vi "XYZStage-Reset axis command.vi"(8 "error in (no error)":errorcluster, 9 "XYZ Stage dequeued data":T2={"Command"=enum."Initialize", "Channel"="Z", "X"=0.0, "Y"=0.0, "Z"=0.0, "Speed"=0, "Zero"=FALSE, "Use acknowledgement?"=TRUE} {"Speed" format="Speed= %.0f"; "Z" format="Z= %#_g"; "Y" format="Y= %#_g"; "X" format="X= %#_g"}, 10 "Z Stage":T1, 11 "XY Stage":T5) -> (0 "error out":errorcluster)   [LabVIEW 2020]
uses:
  Typedefs/XY Stage config cluster.ctl
  Typedefs/XYZ stage data.ctl
  Typedefs/XYZ stage states.ctl
  Typedefs/XYZ channel ring.ctl
  Typedefs/Z Stage config cluster.ctl
  Global Variables/General Globals.vi
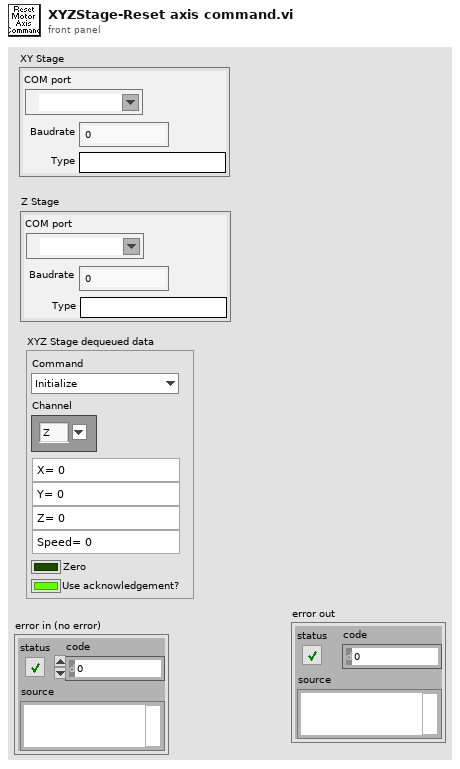
[diagram p1: front panel]
types:
  T1 = typedef "Z Stage config cluster.ctl" = cluster{"COM port":refnum<visa-resource-name>, "Baudrate":i32, "Type":string}
  T2 = typedef "XYZ stage data.ctl" = cluster{"Command":T3, "Channel":T4, "X":sgl, "Y":sgl, "Z":sgl, "Speed":i32, "Zero":bool, "Use acknowledgement?":bool}
  T3 = typedef "XYZ stage states.ctl" = enum16{"Dequeue", "Initialize", "Read Position", "Read Speed Setting", "Move", "Set Max Speed", "Reset Axis", "Stop all movement"}
  T4 = typedef "XYZ channel ring.ctl" = string
  T5 = typedef "XY Stage config cluster.ctl" = cluster{"COM port":refnum<visa-resource-name>, "Baudrate":i32, "Type":string}
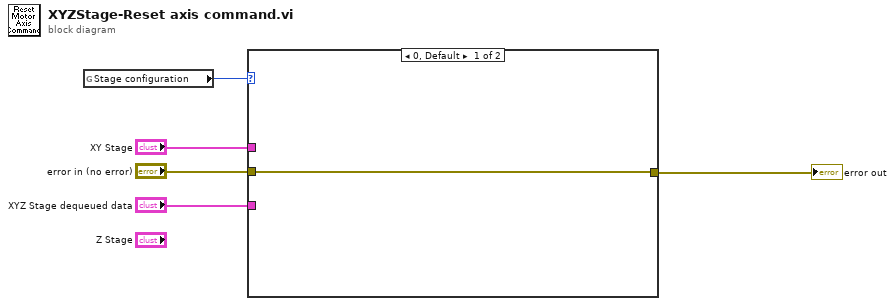
[diagram p0: block diagram]
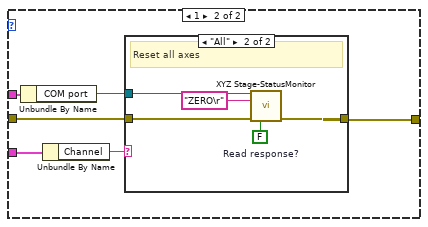
[diagram p2: hidden frame]
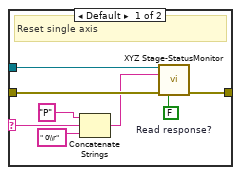
[diagram p3: hidden frame]
diagram:
  n1 = global read "General Globals.vi" "Stage configuration"() -> (w1:i32)
  n2 = case shown="0, Default" w1 {
    tunnel: [w6 w12] -> w5
    tunnel: "XYZ Stage dequeued data" -> [_ w11]
    tunnel: "error in (no error)" -> [w6 w9]
    tunnel: "XY Stage" -> [_ w8]
    frame 0, Default {
    }
    frame 1 {
      n3 = Unbundle By Name(w8) -> ("COM port"=w7:refnum<visa-resource-name>)
      n4 = Unbundle By Name(w11) -> ("Channel"=w10:T4)
      n5 = case shown="\"All\"" w10 {
        selector: w10 -> [w16 _]
        tunnel: w9 -> [w20 w25]
        tunnel: [w15 w24] -> w12
        tunnel: w7 -> [w14 w22]
        frame Default {
          w13 = FALSE  # Read response?
          # "Reset single axis"
          n6 = Concatenate Strings("P" ("string to write"), w16, " 0\\r" ("string")) -> (w17:string)
          n7 = call "XYZ Stage-StatusMonitor.vi"("VISA resource name"=w14, "string to write"=w17, "Error In"=w20, "Read response? (T)"=w13) -> ("Error Out"=w15:errorcluster)  [unwired: 7 in, 4 out]
        }
        frame "All" {
          w21 = FALSE  # Read response?
          # "Reset all axes"
          n8 = call "XYZ Stage-StatusMonitor.vi"("VISA resource name"=w22, "string to write"="ZERO\r", "Error In"=w25, "Read response? (T)"=w21) -> ("Error Out"=w24:errorcluster)  [unwired: 7 in, 4 out]
        }
      }
    }
  }
  "error out" <- w5
